vi "SVXMPL_Set Column Header.vi"(0 "result table":string[][](table), 5 "scaled signals [EU]":waveform(dbl)[](array[waveform]), 11 "error in (no error)":errorcluster) -> (4 "dup result table":string[][](table), 6 "column headers":string[](array[string]), 15 "error out":errorcluster)   [LabVIEW 2017]
doc: "Generates a table based on the results of a fractional-octave analysis."
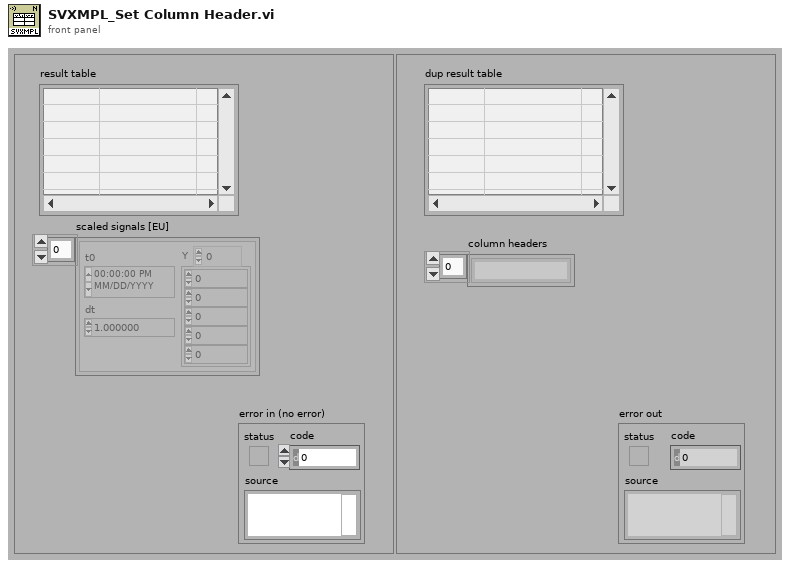
[diagram p1: front panel]
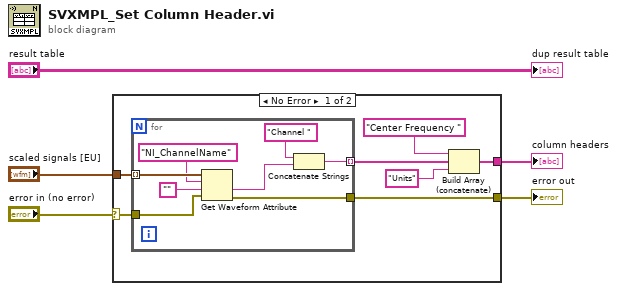
[diagram p0: block diagram]
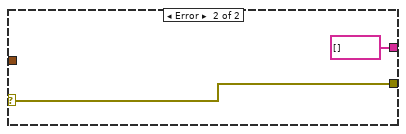
[diagram p2: hidden frame]
diagram:
  n1 = case shown="No Error" "error in (no error)" {
    selector: "error in (no error)" -> [w10 w22]
    tunnel: [w11 w22] -> w2
    tunnel: "scaled signals [EU]" -> [w12 _]
    tunnel: [w6 string[] []] -> w1
    frame No Error {
      n2 = for {
        tunnel: w12 -> [w20] mode=indexing
        tunnel: [w17] -> w11
        tunnel: w10 -> [w16]
        tunnel: [w13] -> w9 mode=indexing
        n3 = Get Waveform Attribute(4:w16, 5:"", 6:"NI_ChannelName" ("name"), 7:w20) -> (0:w17:errorcluster, 1:w15:string)  [unwired: 2 out]
        n4 = Concatenate Strings("Channel " ("name"), w15) -> (w13:string)
      }
      n5 = Build Array (concatenate)("Center Frequency " ("name"), w9, "Units" ("name")) -> (w6:string[])
    }
    frame Error {
    }
  }
  "error out" <- w2
  "column headers" <- w1
  "dup result table" <- "result table"
